vi "ExecLog_WriteToLogFile_Periodic.vi"(3 "error in":errorcluster, 5 "string":string, 6 "FileRef":refnum<file>) -> (0 "error out":errorcluster, 2 "FileRefOut":refnum<file>)   [LabVIEW 2017]
uses:
  LogFileGlobals.vi
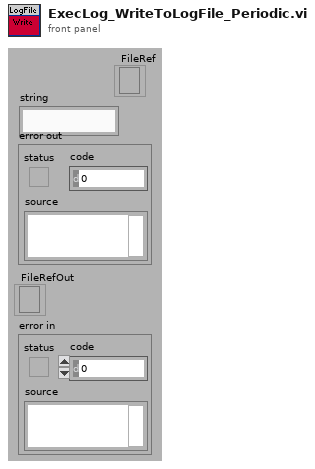
[diagram p1: front panel]
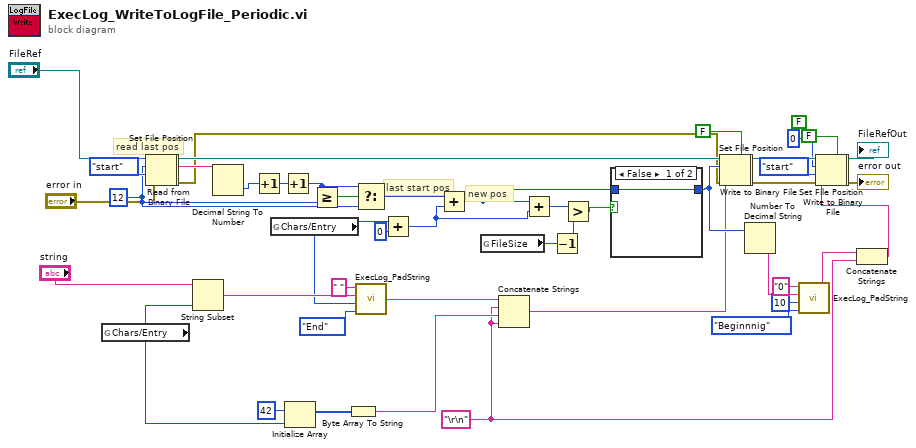
[diagram p0: block diagram]
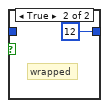
[diagram p2: hidden frame]
diagram:
  (unwired) FALSE ("convert eol (F)")
  w20 = "\r\n" ("string")
  w16 = 12 ("count")
  # "new pos"
  # "read last pos"
  # "last start pos"
  n1 = global read "LogFileGlobals.vi" "Chars/Entry"() -> (w24:u32)
  n2 = Set File Position(refnum="FileRef", from (0:start)=enum16{"start", "end", "current"}."start" ("pos mode (0:2)"), error in="error in") -> (refnum out=w3:refnum<file>, error out=w2:errorcluster)  [unwired: 1 out]
  n3 = Read from Binary File(8:w2, 10:w16, 11:w3) -> (0:w39:errorcluster, 2:w51:string, 3:w50:refnum<file>)  [unwired: 4 out]
  n4 = String Subset(string="string", length (rest)=w24) -> (substring=w29:string)  [unwired: 1 out]
  n5 = Decimal String To Number(string=w51) -> (number=w25:i32)  [unwired: 3 out]
  n6 = Increment(x=w25) -> (x+1=w26:i32)
  n7 = global read "LogFileGlobals.vi" "Chars/Entry"() -> (w18:u32)
  n8 = Increment(x=w26) -> (x+1=w17:i32)
  n9 = Initialize Array(u8 42 ("element"), w24) -> (w22:u8[])
  n10 = Greater Or Equal?(x=w17, y=w16) -> (x >= y?=w33:bool)
  n11 = Byte Array To String(unsigned byte array=w22) -> (string=w21:string)
  n12 = Select(t=w17, s=w33, f=w16) -> (s? t:f=w19:i32)
  n13 = call "ExecLog_PadString.vi"("Location"=enum16{"Beginnnig", "End"}."End", "Length"=w18, "string"=w29, "Pad Character"=" ") -> ("String Out"=w36:string)
  n14 = Add(x=w18, y=u32 0) -> (x+y=w28:u32)
  n15 = Add(x=w19, y=w28) -> (x+y=w43:u32)
  n16 = global read "LogFileGlobals.vi" "FileSize"() -> (w46:u32)
  n17 = Concatenate Strings(w36, w20, w21, w20) -> (w35:string)
  n18 = Add(x=w43, y=w28) -> (x+y=w47:u32)
  n19 = Decrement(x=w46) -> (x-1=w45:u32)
  n20 = Greater?(x=w47, y=w45) -> (0:w44:bool)
  n21 = case shown="False" w44 {
    tunnel: [w53 u32 12] -> w41
    tunnel: w43 -> [w53 _]
    frame False {
    }
    frame True {
      # "wrapped"
    }
  }
  n22 = Set File Position(offset (in bytes) (0)=w41, refnum=w50, error in=w39) -> (refnum out=w6:refnum<file>, error out=w5:errorcluster)  [unwired: 1 out]
  n23 = Write to Binary File(file (use dialog)=w6, data=w35, error in=w5, 5:FALSE ("prepend array or string size? (T)")) -> (refnum out=w42:refnum<file>, error out=w40:errorcluster)  [unwired: 3 out]
  n24 = Number To Decimal String(number=w41) -> (decimal integer string=w13:string)  [unwired: 1 out]
  n25 = call "ExecLog_PadString.vi"("Location"=enum16{"Beginnnig", "End"}."Beginnnig", "Length"=10, "string"=w13, "Pad Character"="0") -> ("String Out"=w11:string)
  n26 = Set File Position(offset (in bytes) (0)=0 ("pos offset (0)"), refnum=w42, from (0:start)=enum16{"start", "end", "current"}."start" ("pos mode (0:2)"), error in=w40) -> (refnum out=w9:refnum<file>, error out=w8:errorcluster)
  n27 = Concatenate Strings(w11, w20) -> (w31:string)
  n28 = Write to Binary File(file (use dialog)=w9, data=w31, error in=w8, 5:FALSE ("prepend array or string size? (T)")) -> (refnum out=→"FileRefOut":refnum<file>, error out=→"error out":errorcluster)  [unwired: 3 out]
